vi "Szybka na wysw FVG.vi"(6 "Restart in":bool, 7 "Akcja (GET)":T2, 8 "error in (no error)":errorcluster, 9 "Bufor in":T1, 10 "Czas in":i32, 11 "Œledzenie in":enum16{"Obwiednia", "Migawka"}(ring)) -> (0 "error out":errorcluster, 1 "Œledzenie out":enum16{"Obwiednia", "Migawka"}(ring), 2 "Bufor out":T1, 3 "Czas Out":i32, 4 "Restart out":bool)   [LabVIEW 2013]
doc: "Use this template to build a VI to use as a subVI."
uses:
  Kontrolki/FVGs/FVG akcje podstawowa.ctl
  Kontrolki/Przetwarzanie/Kanaly.ctl
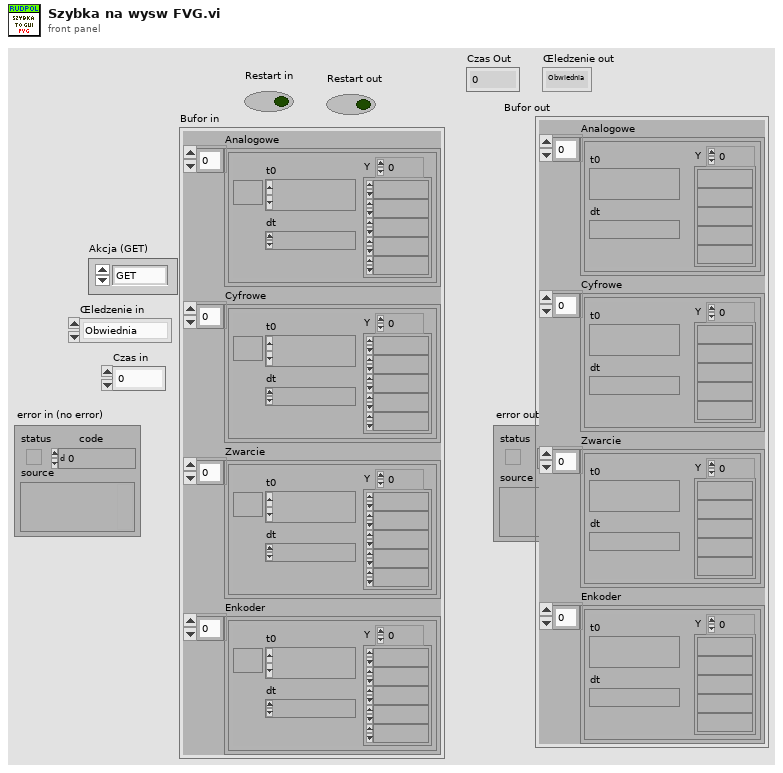
[diagram p1: front panel]
types:
  T1 = typedef "Kanaly.ctl" = cluster{"Analogowe":waveform(dbl)[], "Cyfrowe":waveform(dbl)[], "Zwarcie":waveform(dbl)[], "Enkoder":waveform(dbl)[]}
  T2 = typedef "FVG akcje podstawowa.ctl" = enum16{"GET", "SET"}
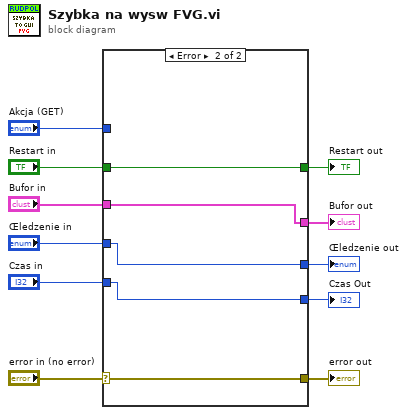
[diagram p0: block diagram]
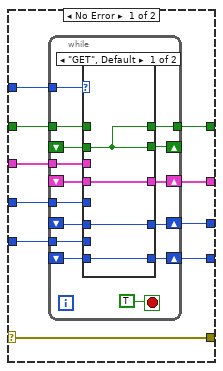
[diagram p2: hidden frame]
diagram:
  n1 = case shown="Error" "error in (no error)" {
    selector: "error in (no error)" -> [w21 w49]
    tunnel: [w21 w49] -> w10
    tunnel: "Akcja (GET)" -> [w20 _]
    tunnel: "Czas in" -> [w19 w48]
    tunnel: "Œledzenie in" -> [w18 w47]
    tunnel: "Bufor in" -> [w17 w46]
    tunnel: [w16 w48] -> w5
    tunnel: [w15 w47] -> w4
    tunnel: [w14 w46] -> w3
    tunnel: "Restart in" -> [w13 w45]
    tunnel: [w12 w45] -> w1
    frame No Error {
      n2 = while {
        tunnel: w20 -> [w35]
        tunnel: w19 -> [w34]
        tunnel: w18 -> [w33]
        tunnel: w17 -> [w32]
        shift-right: [w31] -> w14
        shift-left: _ -> [w30]
        shift-right: [w29] -> w15
        shift-left: _ -> [w28]
        shift-right: [w27] -> w16
        shift-left: _ -> [w26]
        tunnel: w13 -> [w25]
        shift-right: [w24] -> _
        shift-left: _ -> [w22]
        tunnel: [w23] -> w12
        stop <- TRUE stop-if-true
        n3 = case shown="\"GET\", Default" w35 {
          tunnel: w34 -> [_ w42]
          tunnel: w33 -> [_ w43]
          tunnel: w32 -> [_ w44]
          tunnel: [w40 w44] -> w31
          tunnel: w30 -> [w40 _]
          tunnel: [w39 w43] -> w29
          tunnel: w28 -> [w39 _]
          tunnel: [w38 w42] -> w27
          tunnel: w26 -> [w38 _]
          tunnel: w25 -> [_ w41]
          tunnel: [w37 w41] -> w24
          tunnel: [w37 w41] -> w23
          tunnel: w22 -> [w37 _]
          frame "GET", Default {
          }
          frame "SET" {
          }
        }
      }
    }
    frame Error {
    }
  }
  "error out" <- w10
  "Czas Out" <- w5
  "Bufor out" <- w3
  "Œledzenie out" <- w4
  "Restart out" <- w1
